vi "test.vi"() -> ()   [LabVIEW 2014]
uses:
  Robot2015.xctl
panel:
  in  "Opening":enum16{"Close", "Narrow", "Wide"}(ring)
  in  "stop":bool
  in  "position":dbl
  out "Robot2015":dbl(xcontrol)
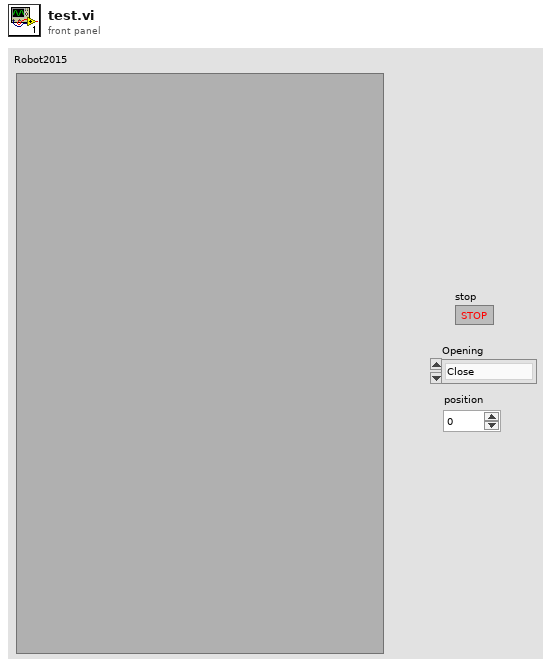
[diagram p1: front panel]
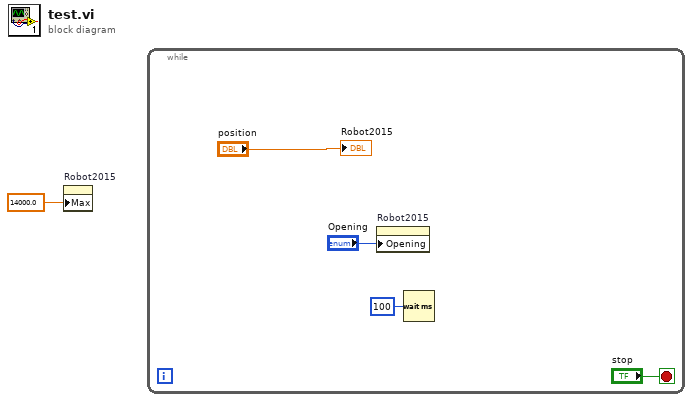
[diagram p0: block diagram]
diagram:
  n1 = property on="Robot2015" class="Robot2015 (strict)"("Max"=14000.0) -> ()  [unwired: 2 in, 2 out]
  n2 = while {
    stop <- "stop" stop-if-true
    n3 = property on="Robot2015" class="Robot2015 (strict)"("Opening"="Opening") -> ()  [unwired: 2 in, 2 out]
    n4 = Wait (ms)(milliseconds to wait=u32 100) -> ()  [unwired: 1 out]
    "Robot2015" <- "position"
  }
